vi "Display Resultado.vi"(8 "error in (no error)":errorcluster, 11 "Calculadora in":refnum<class "Calculadora.lvclass">) -> (0 "error out":errorcluster, 3 "Calculadora out":refnum<class "Calculadora.lvclass">)   [LabVIEW 2020, in "Calculadora.lvlib" / "Calculadora.lvclass"]
uses:
  Calculadora.lvclass
  Calculadora.lvclass/Calculadora.ctl
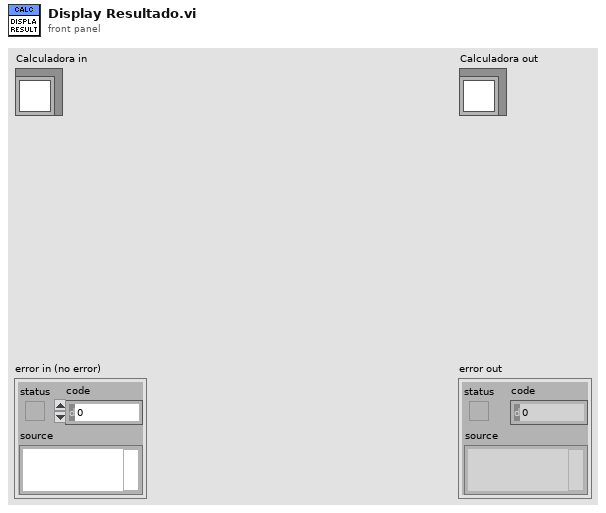
[diagram p1: front panel]
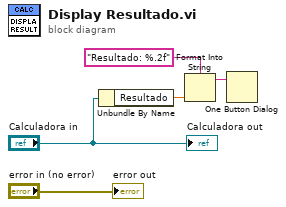
[diagram p0: block diagram]
diagram:
  n1 = Unbundle By Name("Calculadora in") -> ("Resultado"=w3:dbl)
  n2 = Format Into String(format string="Resultado: %.2f", w3) -> (resulting string=w2:string)  [unwired: 2 in, 1 out]
  n3 = One Button Dialog(message=w2) -> ()  [unwired: 1 in, 1 out]
  "error out" <- "error in (no error)"
  "Calculadora out" <- "Calculadora in"
